vi "Schrödinger's Cat.vi"(8 "error in (no error)":errorcluster) -> (0 "error out":errorcluster, 2 "Boolean":bool)   [LabVIEW 2020]
uses:
  <vilib>/Utility/error.llb/Error Cluster From Error Code.vi
  <vilib>/ErrorRing/Error Ring.xnode
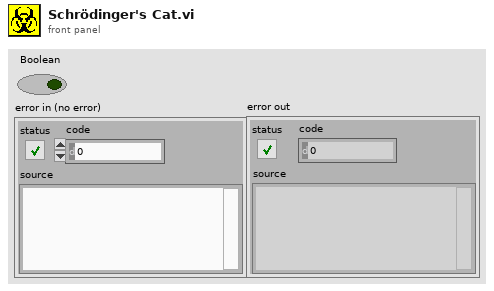
[diagram p1: front panel]
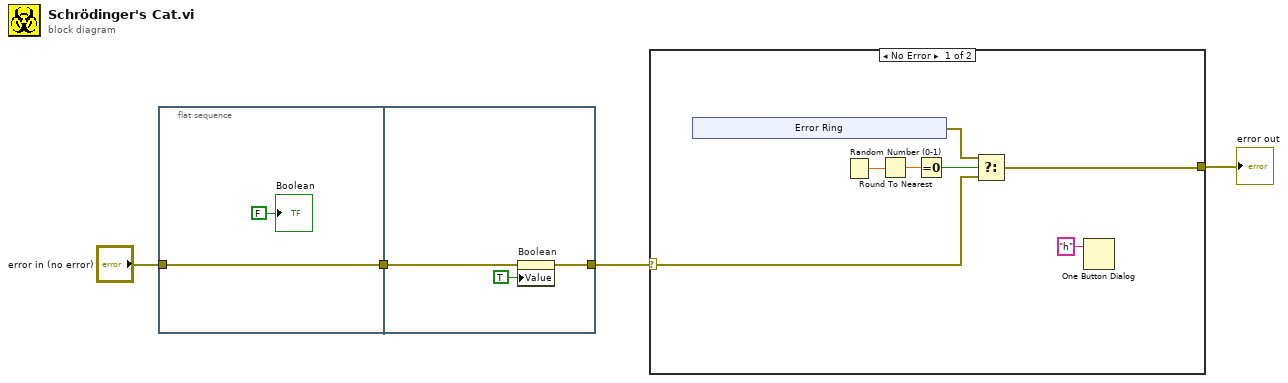
[diagram p0: block diagram]
diagram:
  n1 = flat-sequence {
    tunnel: "error in (no error)" -> [w6]
    tunnel: [w6] -> w1
    tunnel: [w8] -> w2
    tunnel: w1 -> [w9]
    frame #0 {
      "Boolean" <- FALSE ("Boolean")
    }
    frame #1 {
      n2 = property on="Boolean" class="Bool (strict)"(error in=w9, "Value"=TRUE ("Boolean")) -> (error out=w8:errorcluster)  [unwired: 1 in, 1 out]
    }
  }
  n3 = case shown="No Error" w2 {
    selector: w2 -> [w10 w21]
    tunnel: [w11 w21] -> w4
    frame No Error {
      n4 = xnode "Error Ring"() -> ("error out"=w13:errorcluster)
      n5 = Random Number (0-1)() -> (number: 0 to 1=w16:dbl)
      n6 = Round To Nearest(number=w16) -> (nearest integer value=w15:dbl)
      n7 = Equal To 0?(x=w15) -> (x = 0?=w14:bool)
      n8 = Select(t=w13, s=w14, f=w10) -> (s? t:f=w11:errorcluster)
      n9 = One Button Dialog(message="h") -> ()  [unwired: 1 in, 1 out]
    }
    frame Error {
    }
  }
  "error out" <- w4
